vi "ORP电极校准.vi"() -> ()   [LabVIEW 2016, in "斯坦道多参数.lvlib"]
uses:
  <vilib>/Utility/miscctls.llb/LVPointTypeDef.ctl
  <vilib>/Analysis/NI_AALBase.lvlib
  <vilib>/Utility/config.llb/NI_LVConfig.lvlib
panel:
  out "滤波设定":dbl
  in  "刷新按钮":bool
  out "第二点信号值":dbl
  out "第一点信号值":dbl
  out "通讯状态":string
  out "温度":dbl format="%#.2f"
  out "当前信号值":dbl caption="信号值" format="%#.2f"
  in  "校准停止":bool
  in  "校准启动":bool
  out "波形图表":sgl(graph) caption="历史曲线"
  out "第二点校准值":dbl
  out "第一点校准值":dbl
  in  "校准模式":u16(ring) items=["单点校准"]
  out "提示":string
  out "最小值":sgl format="%#.2f"
  out "最大值":sgl format="%#.2f"
  out "mean":dbl caption="均值" format="%#.2f"
  out "standard deviation":dbl caption="标准差" format="%#.2f"
  out "变异系数":dbl format="%#.6f"
  in  "标液1":dbl
  out "当前读取值":dbl caption="测量值" format="%#.2f"
  out "ORP偏移修正值":dbl format="%#.2f"
  # "ORP电极设定"
  # "请选择校准模式:"
  # "℃"
  # "mV"
  # "mV"
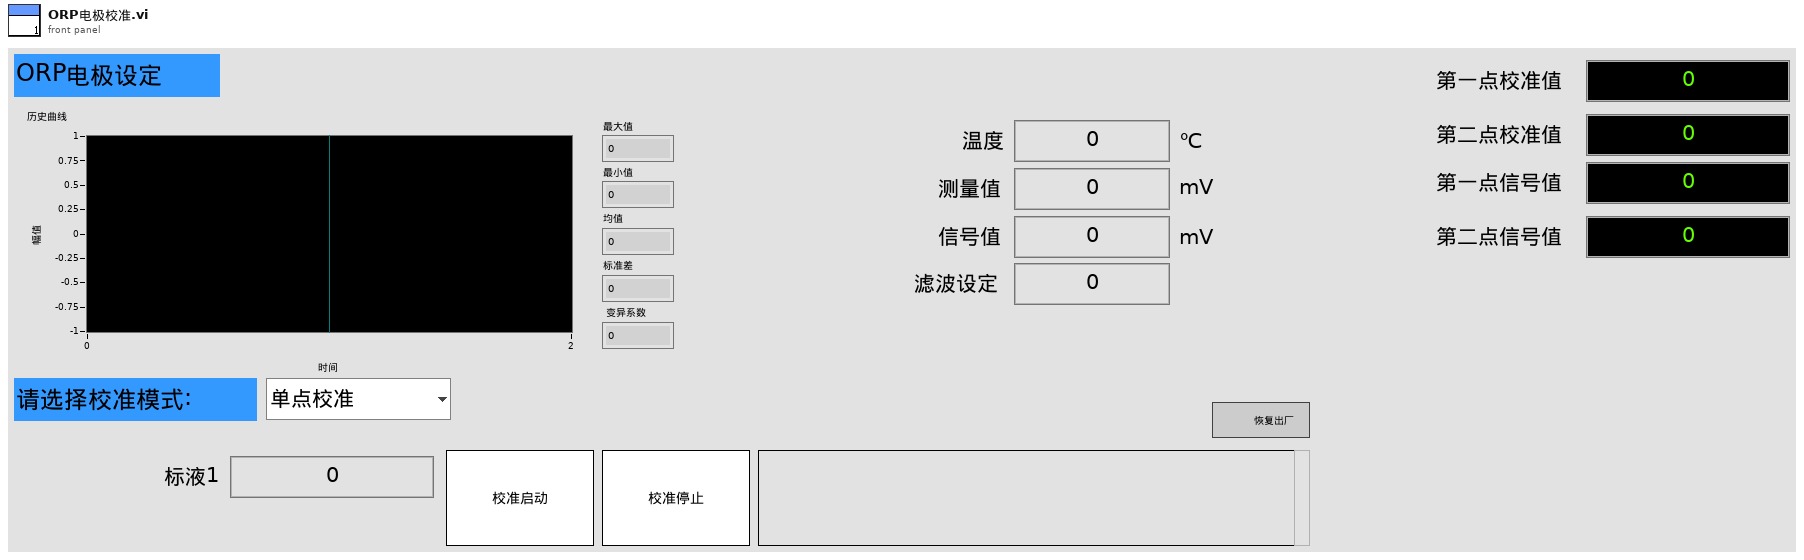
[diagram p1: front panel]
types:
  T1 = typedef "斯坦道多参数.lvlib/通知队列类型.ctl" = enum16{"pH", "DO", "Cond", "Turb", "ORP", "叶绿素a", "藻密度", "COD"}
  T2 = typedef "LVPointTypeDef.ctl" = cluster{"Horizontal":i16, "Vertical":i16}
  T3 = typedef "NI_LVConfig.lvlib/Config Data RefNum.ctl" = refnum<k1>
  T4 = cluster{"电极状态标志":u16, "电极型号标志":u16, "测量值":sgl, "温度测量值":sgl, "信号值":sgl, "温度信号值":sgl, "000AH_NC":sgl, "偏移修正值":sgl, "温度偏移修正值":sgl, "手动温度补偿值":sgl, "命令滤波设定":u16, "温度模式":enum16{"ATC", "MTC"}, "生产批次":u16, "传感器序号":u16, "串口地址":u16, "串口波特率":enum16{"9600", "19200", "115200"}, "串口校验位":enum16{"NONE", "ODD", "EVEN"}, "串口停止位":enum16{"1bit", "2bit"}}
  T5 = enum16{"pH", "DO", "Cond", "Turb", "ORP", "叶绿素a", "藻密度"}
  T6 = enum8{"Enabled", "Disabled", "Disabled and Grayed Out"}
  T7 = cluster{"ph":bool, "DO":bool, "Cond":bool, "Turb":bool, "叶绿素a":bool, "藻密度":bool, "ORP":bool, "COD":bool}
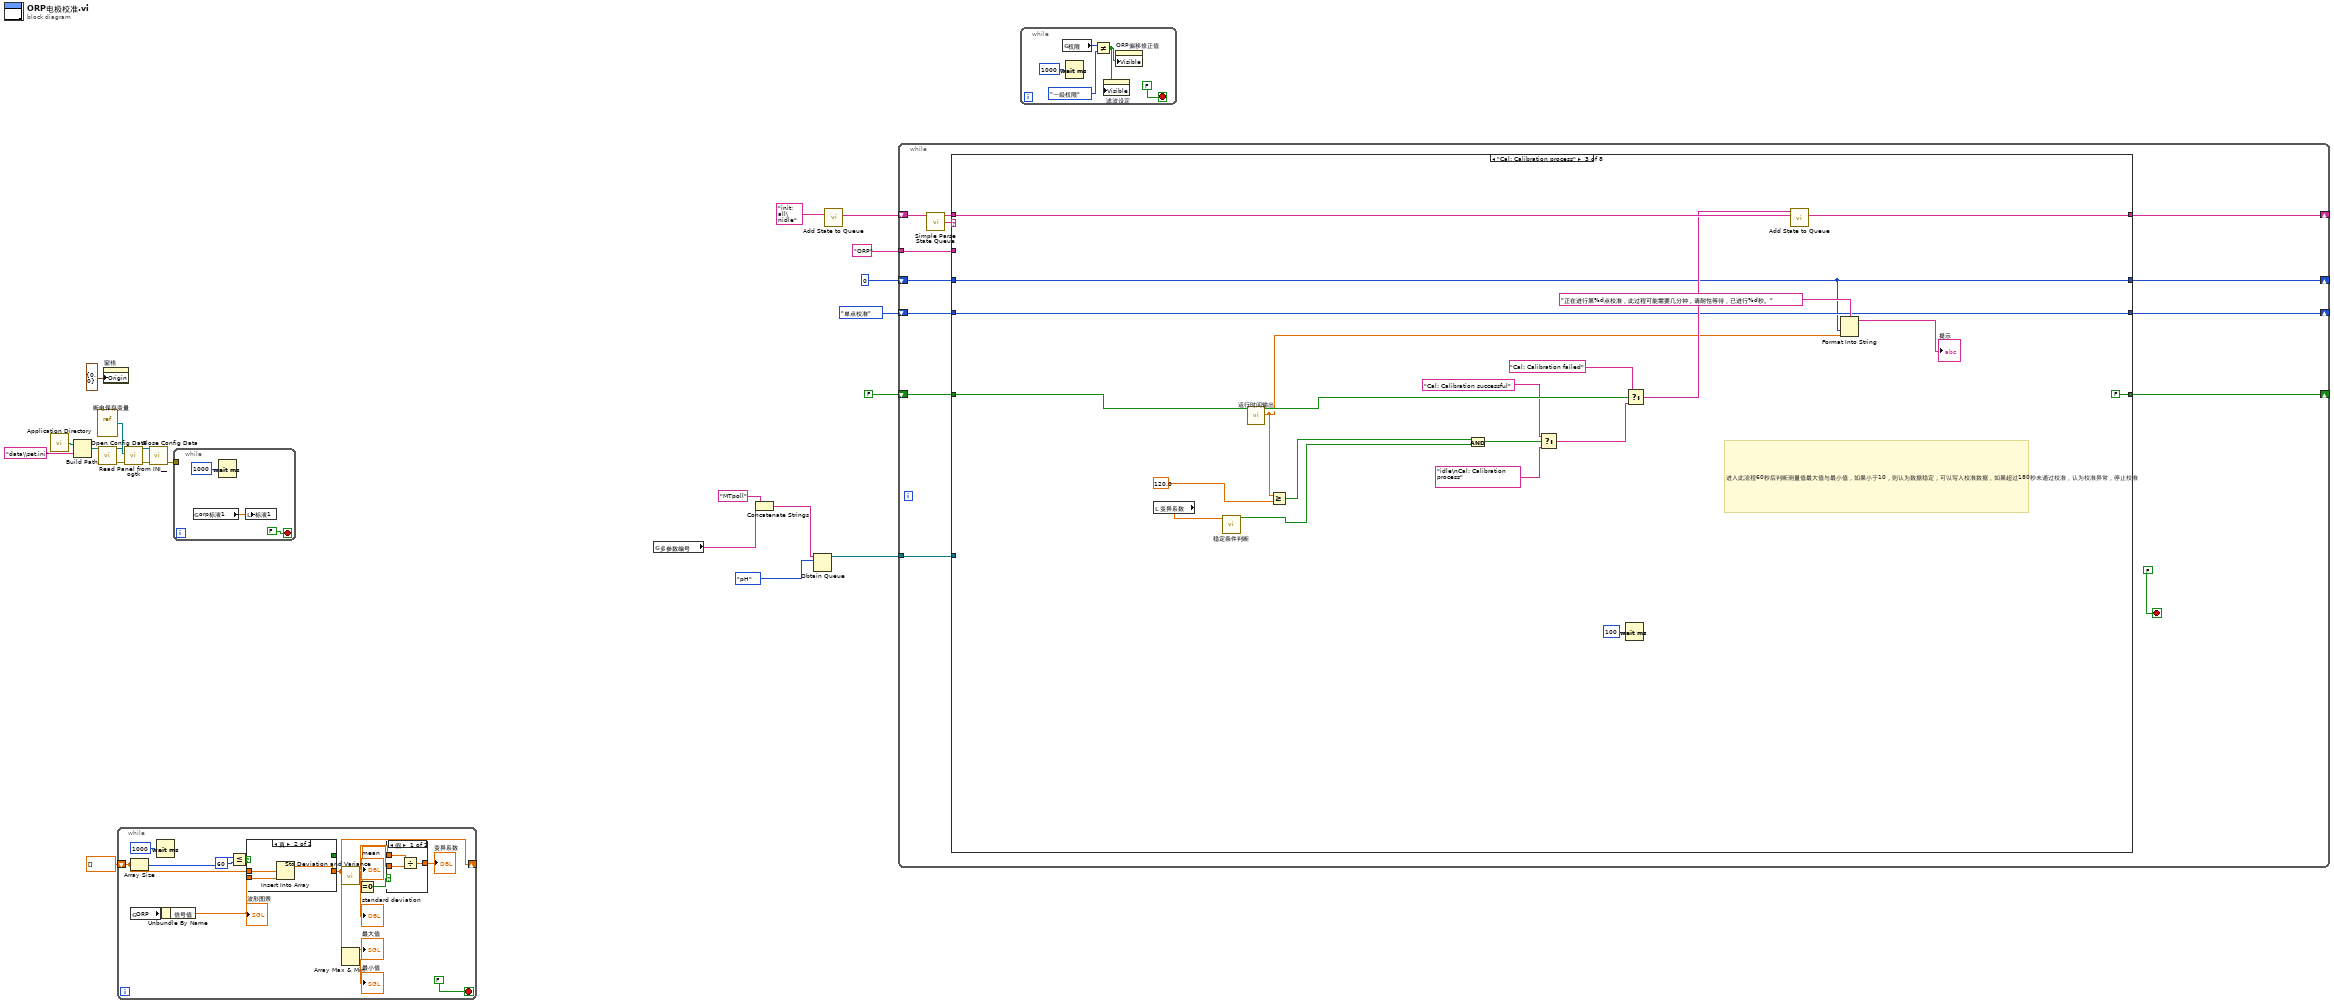
[diagram p0: block diagram]
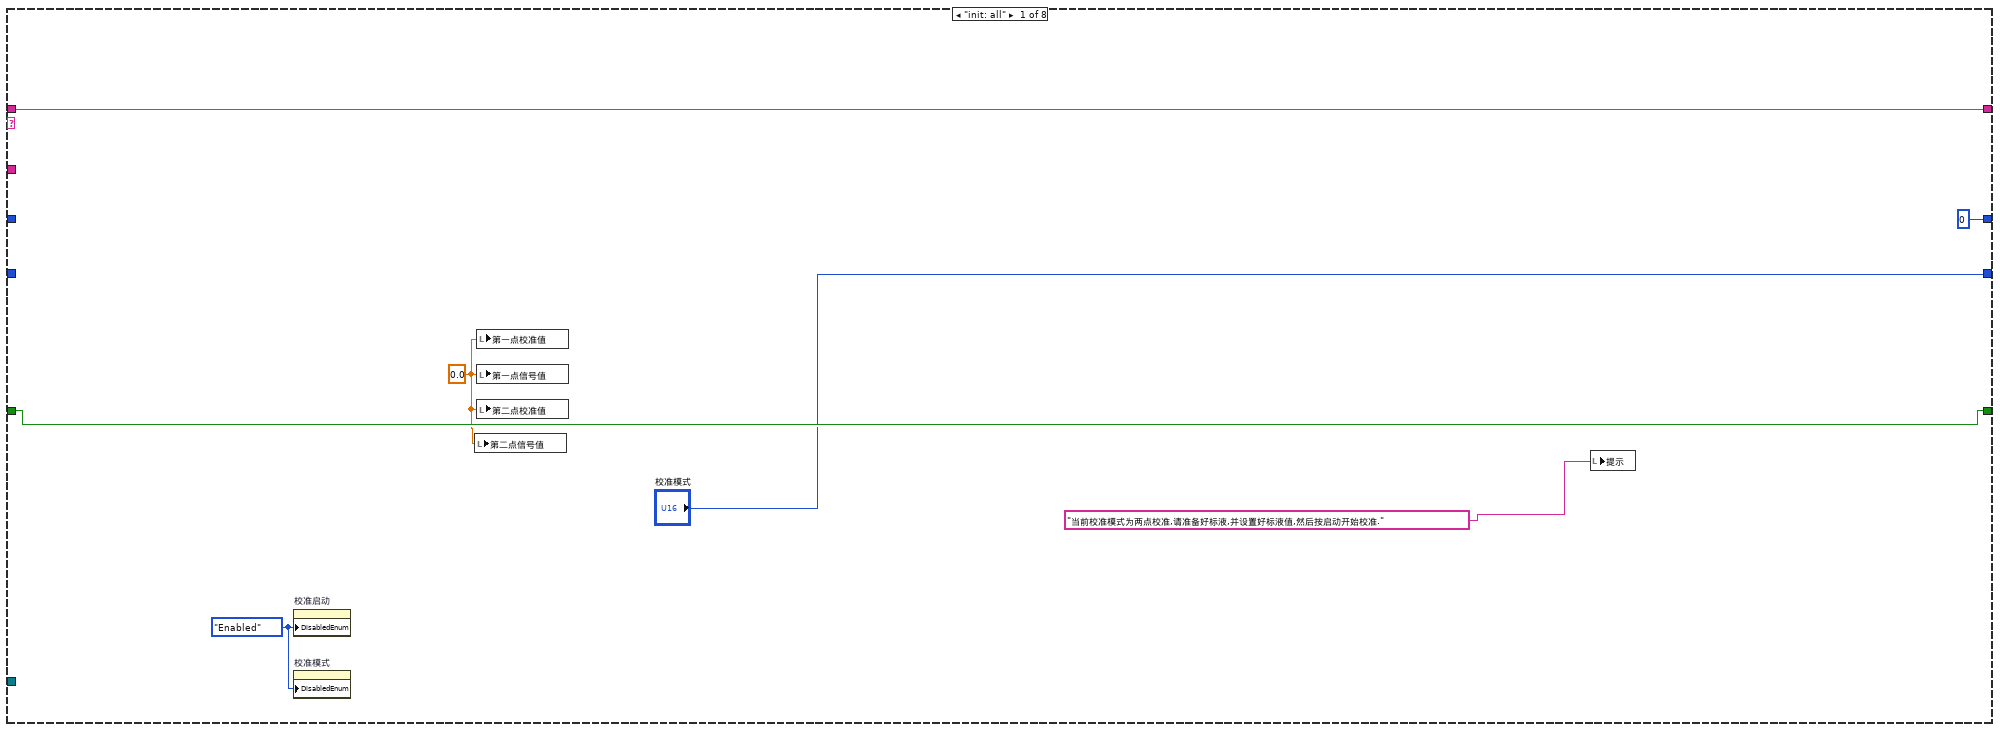
[diagram p2: hidden frame]
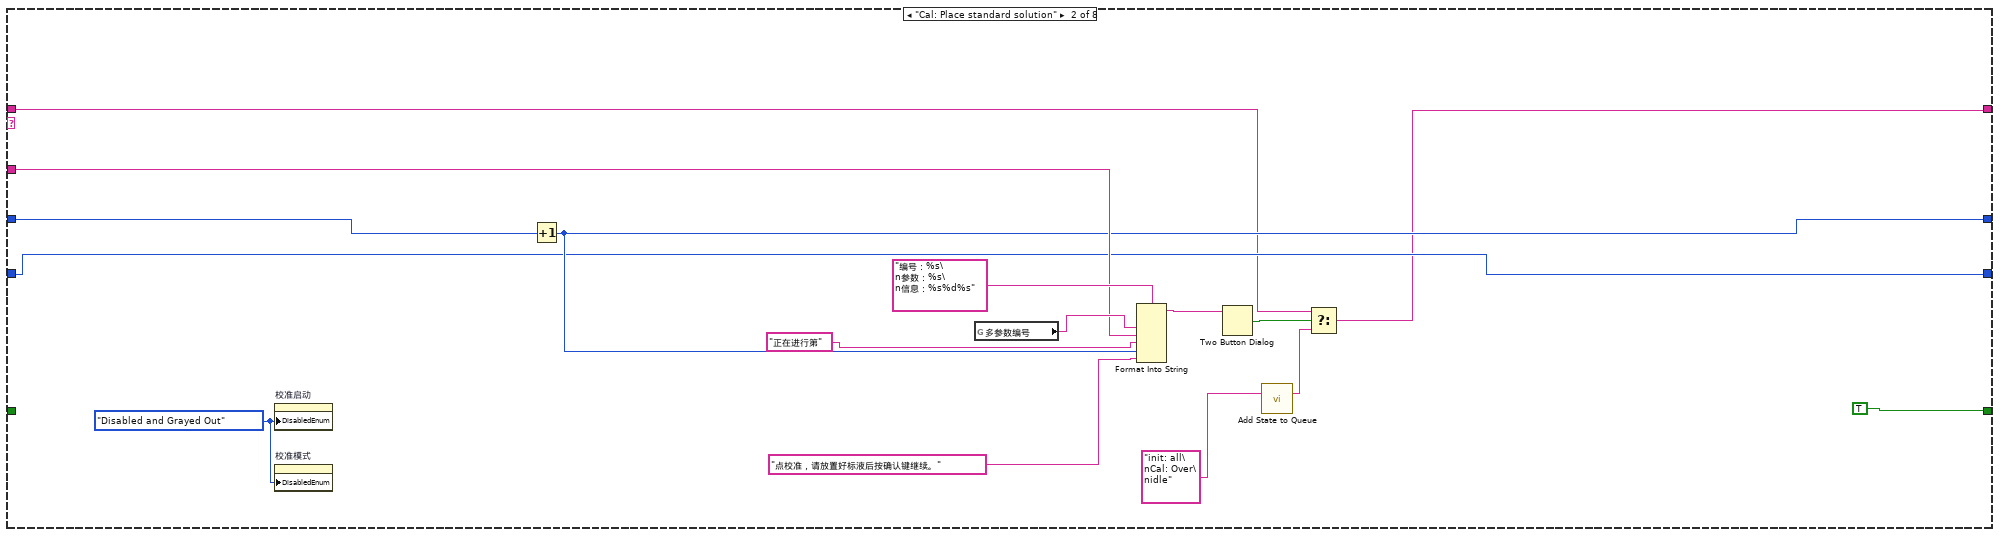
[diagram p3: hidden frame]
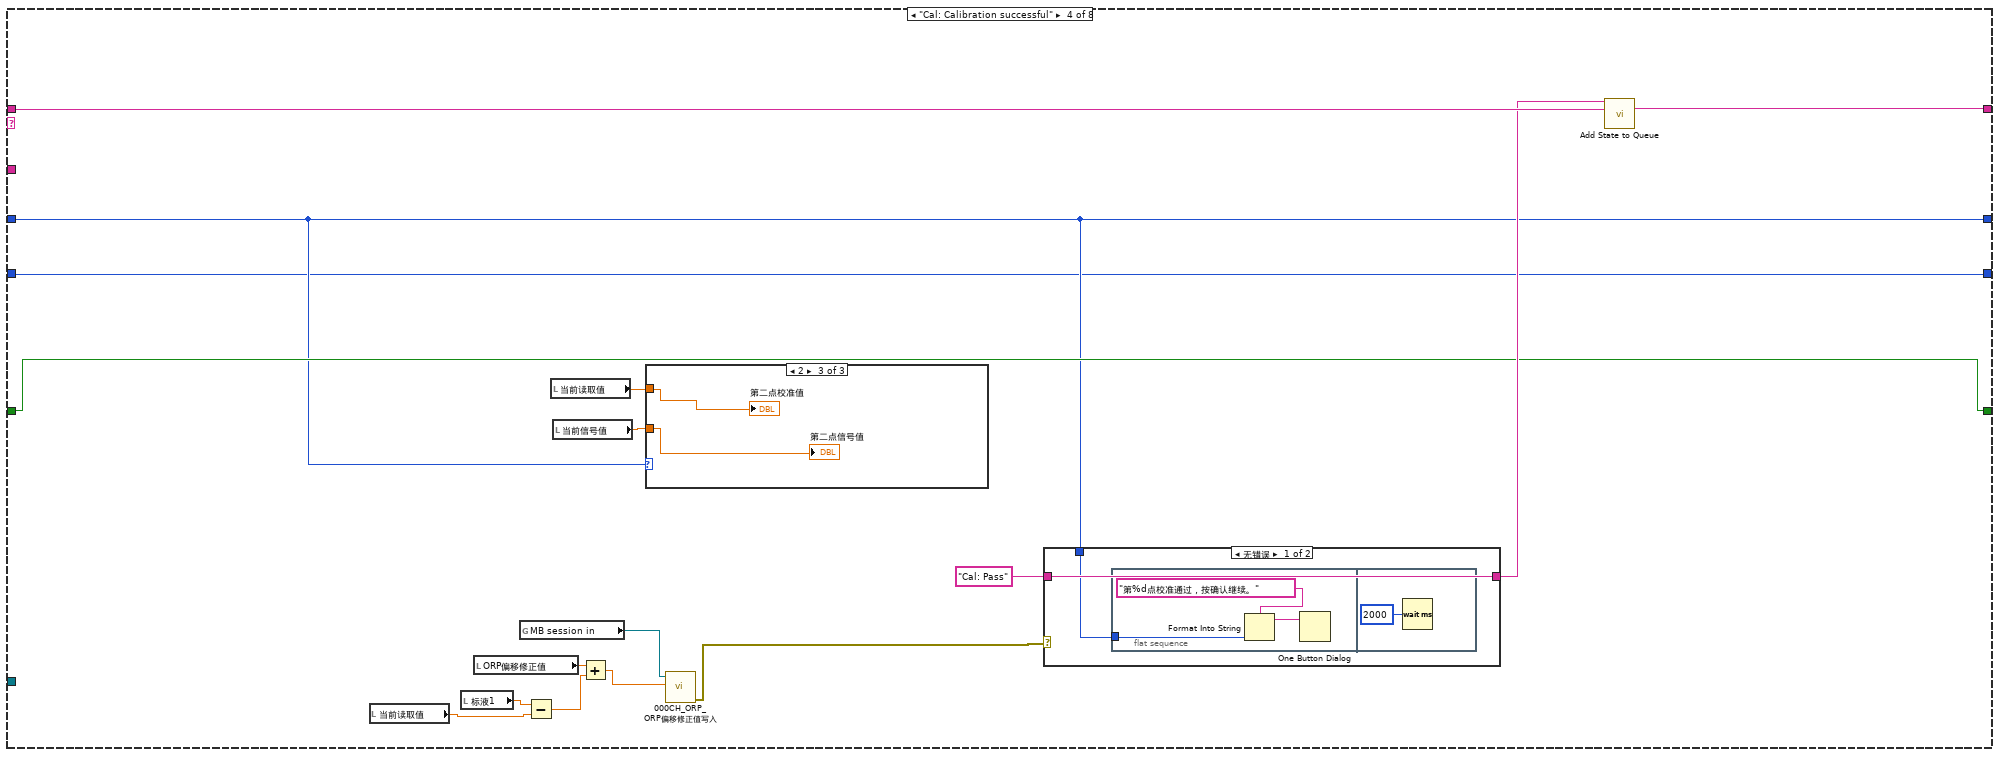
[diagram p4: hidden frame]
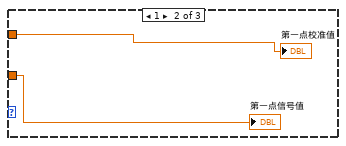
[diagram p6: hidden frame]
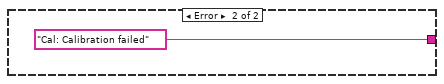
[diagram p7: hidden frame]
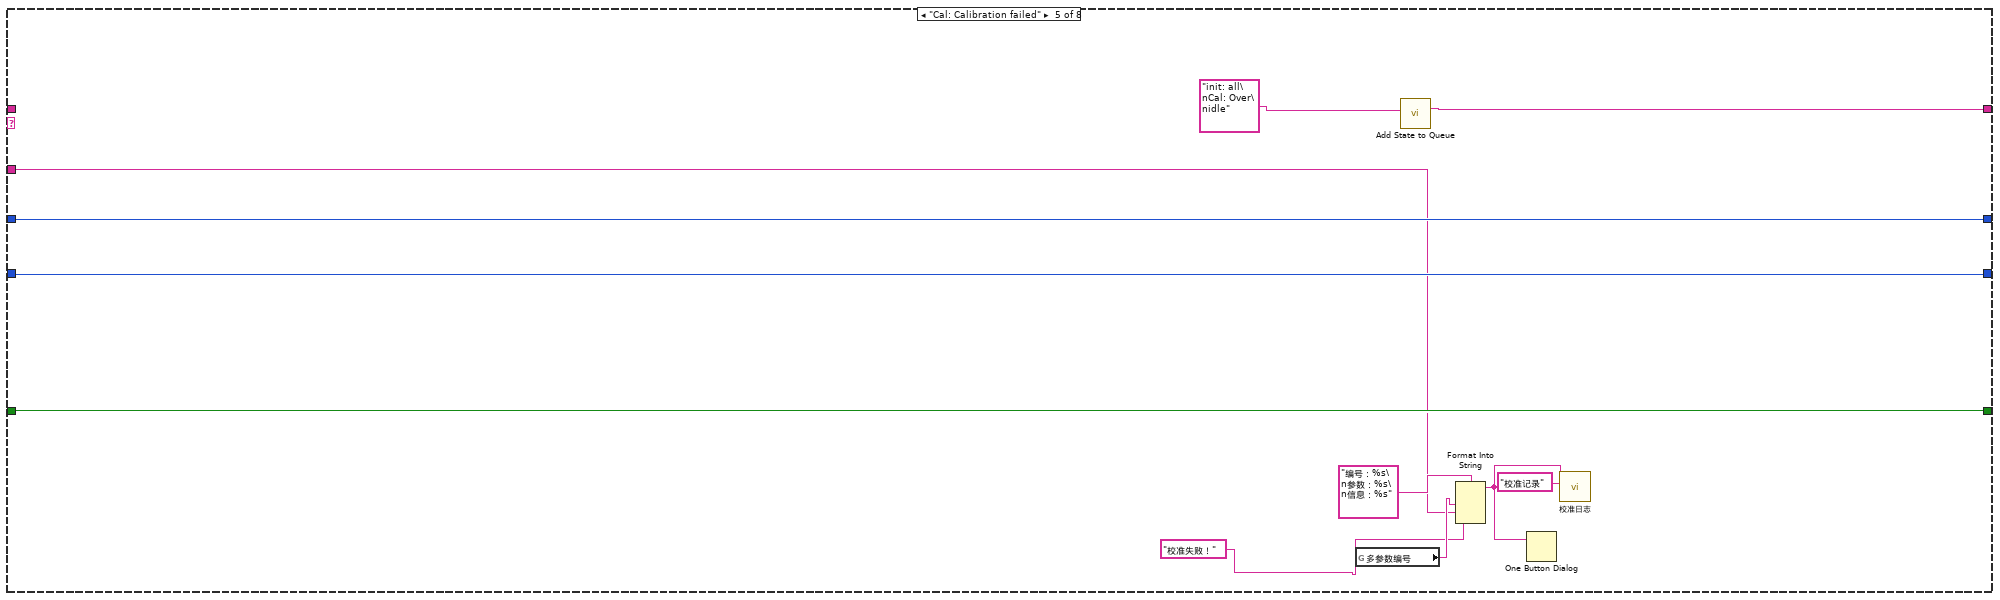
[diagram p8: hidden frame]
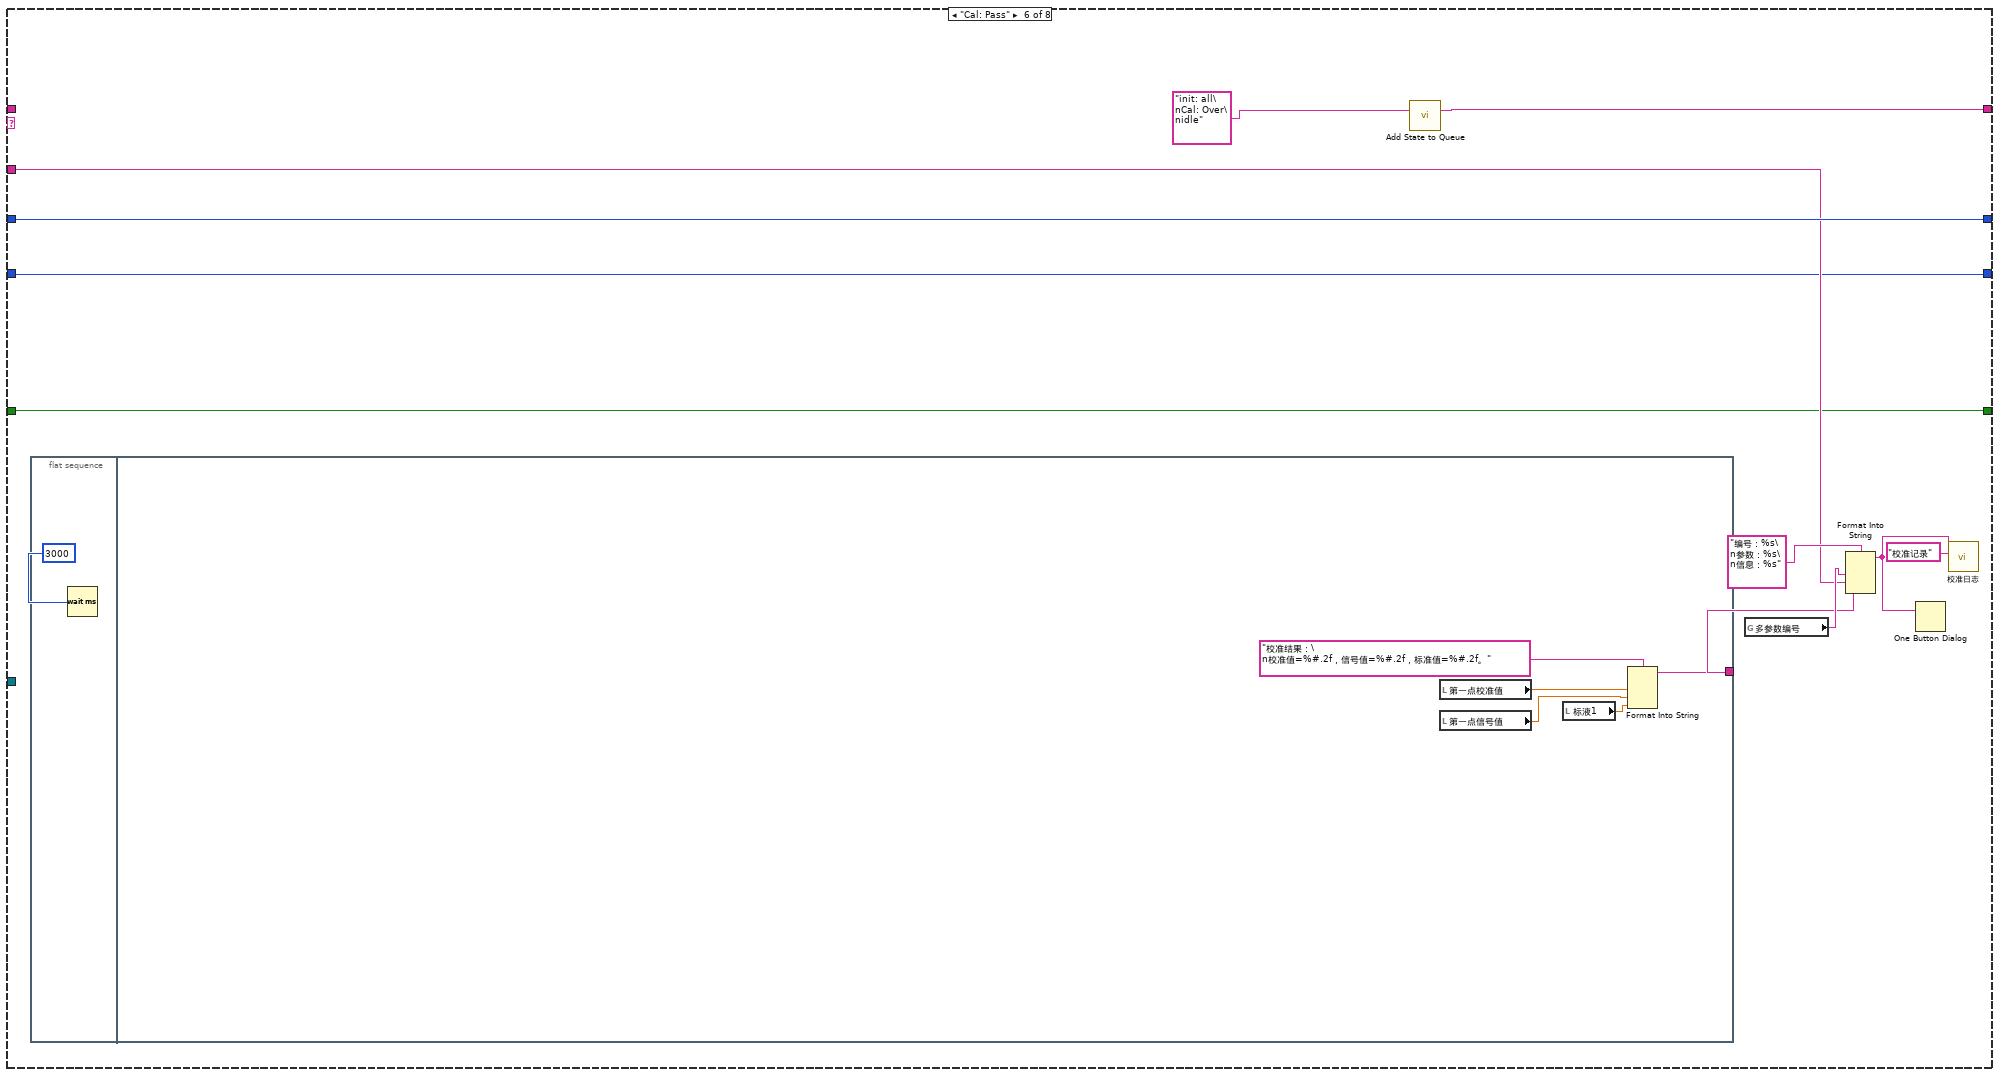
[diagram p9: hidden frame]
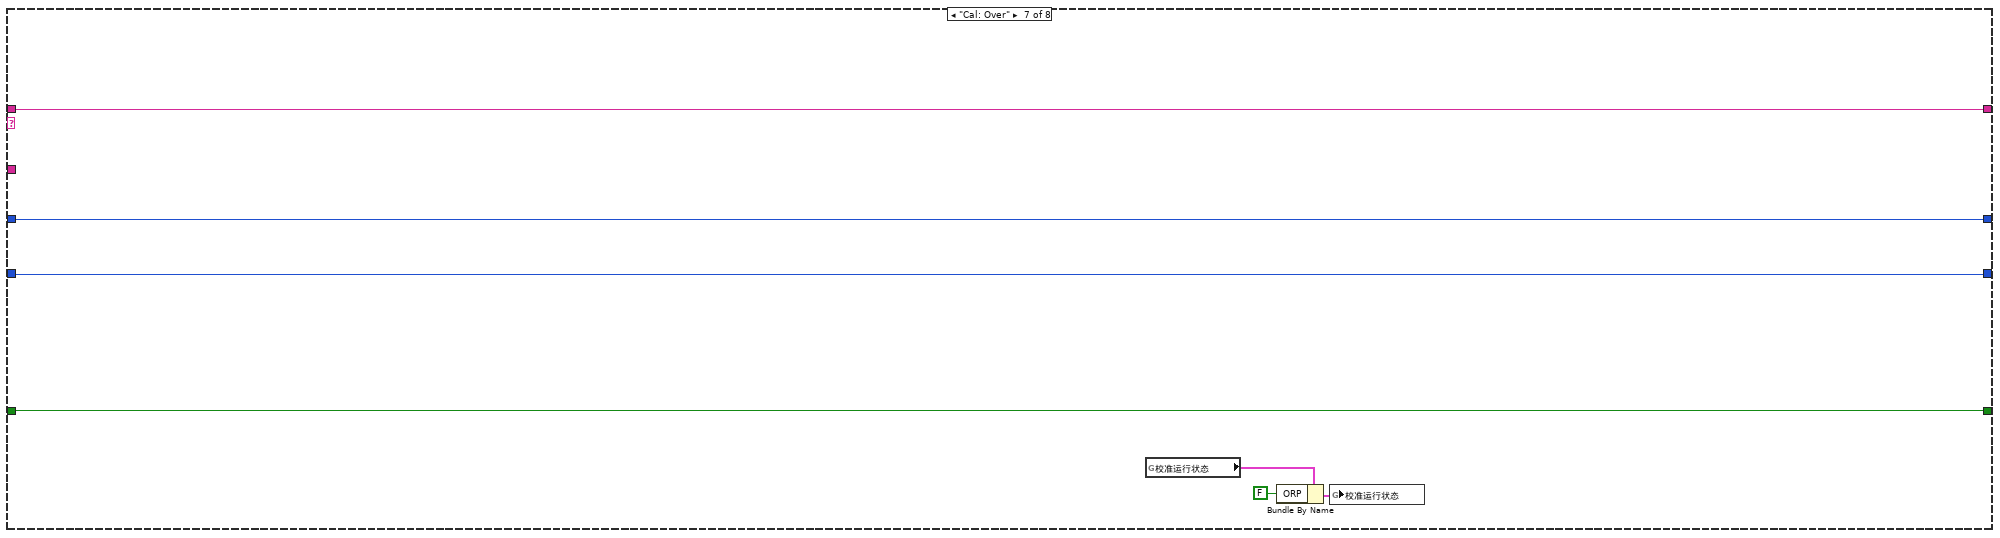
[diagram p10: hidden frame]
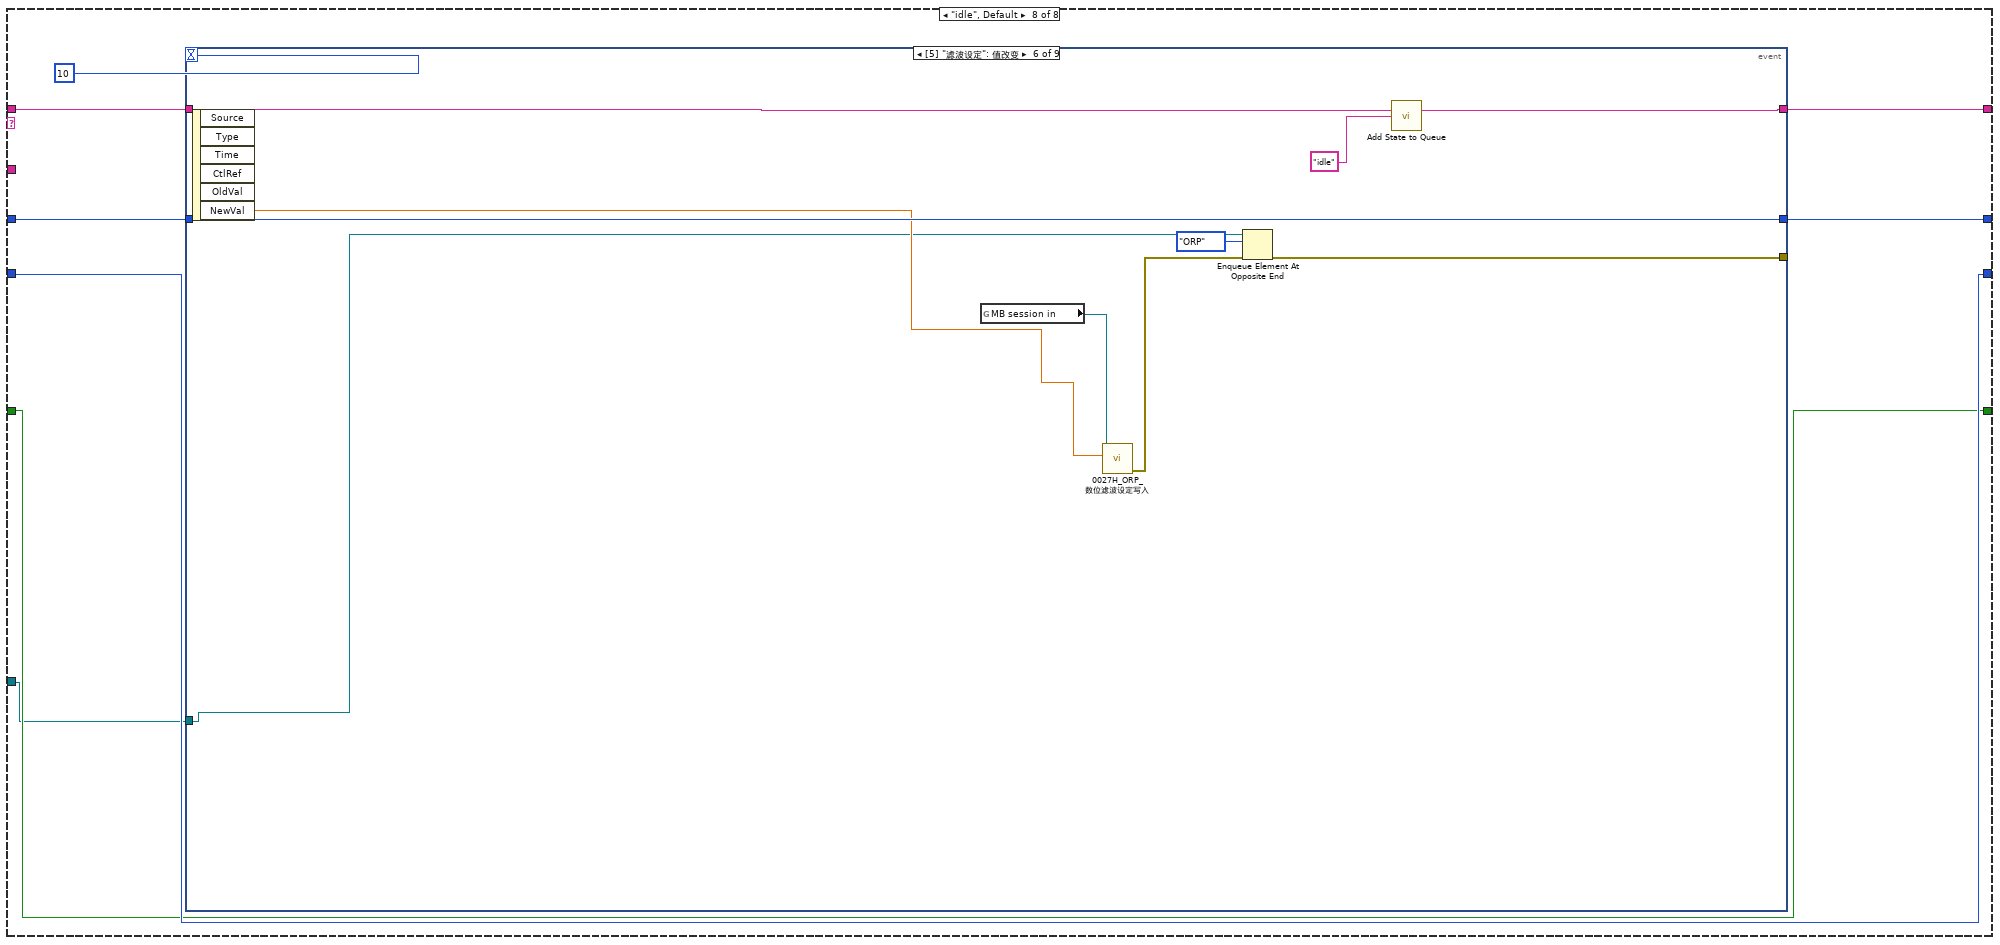
[diagram p11: hidden frame]
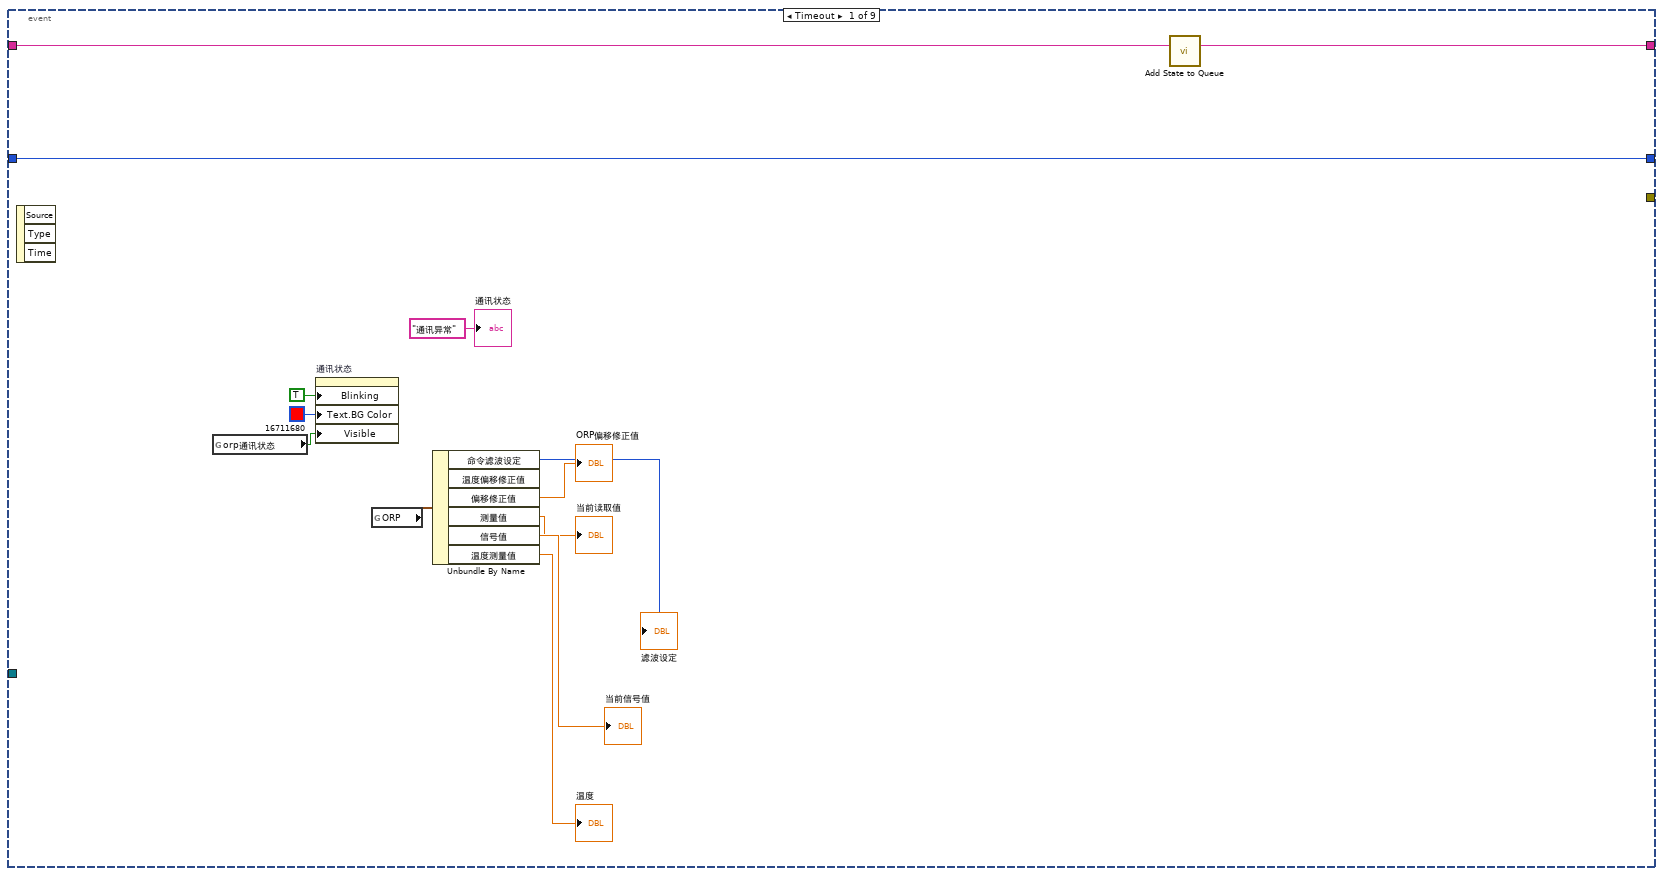
[diagram p12: hidden frame]
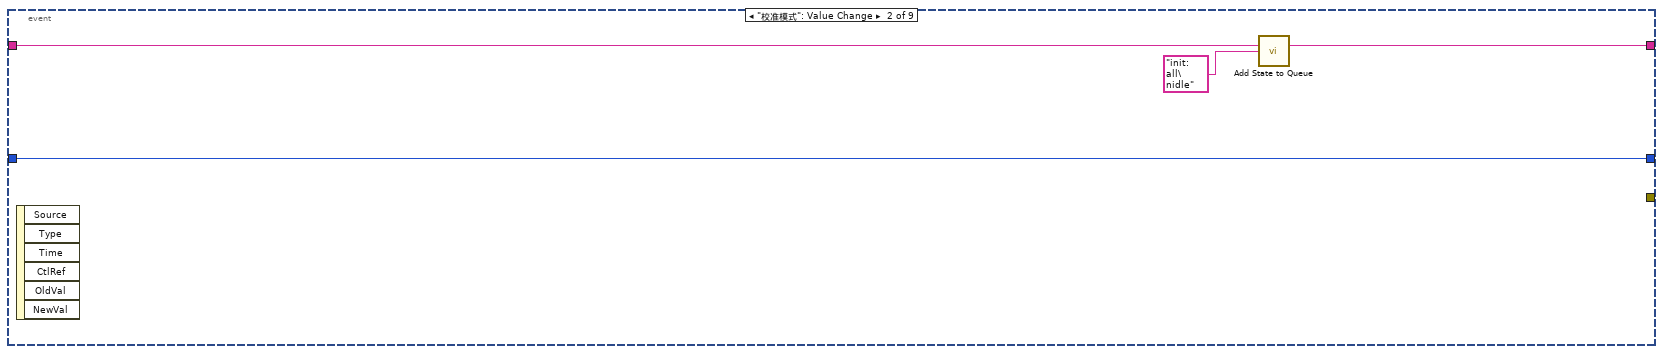
[diagram p13: hidden frame]
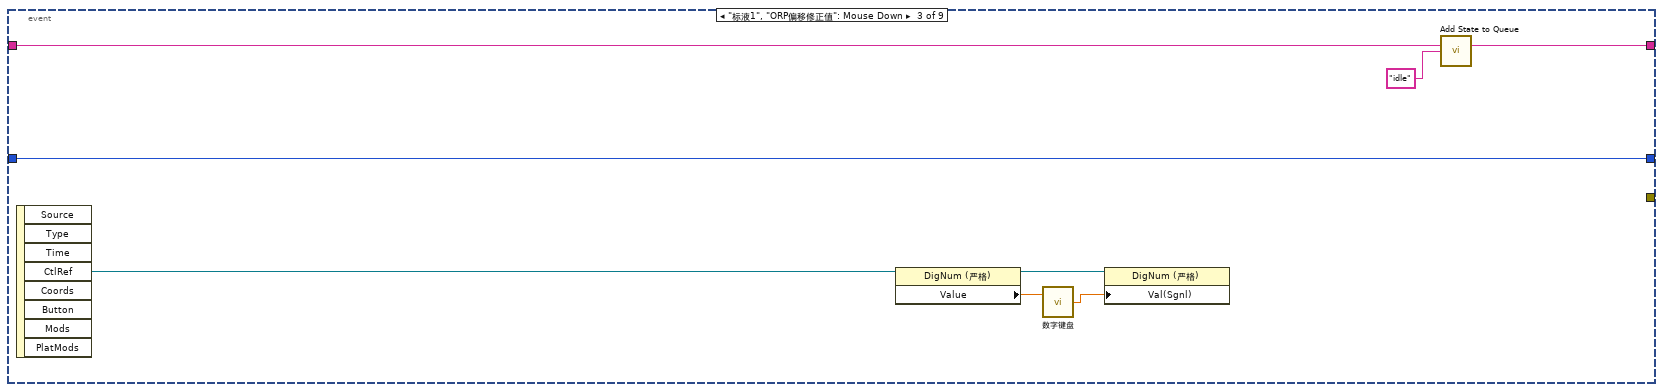
[diagram p14: hidden frame]
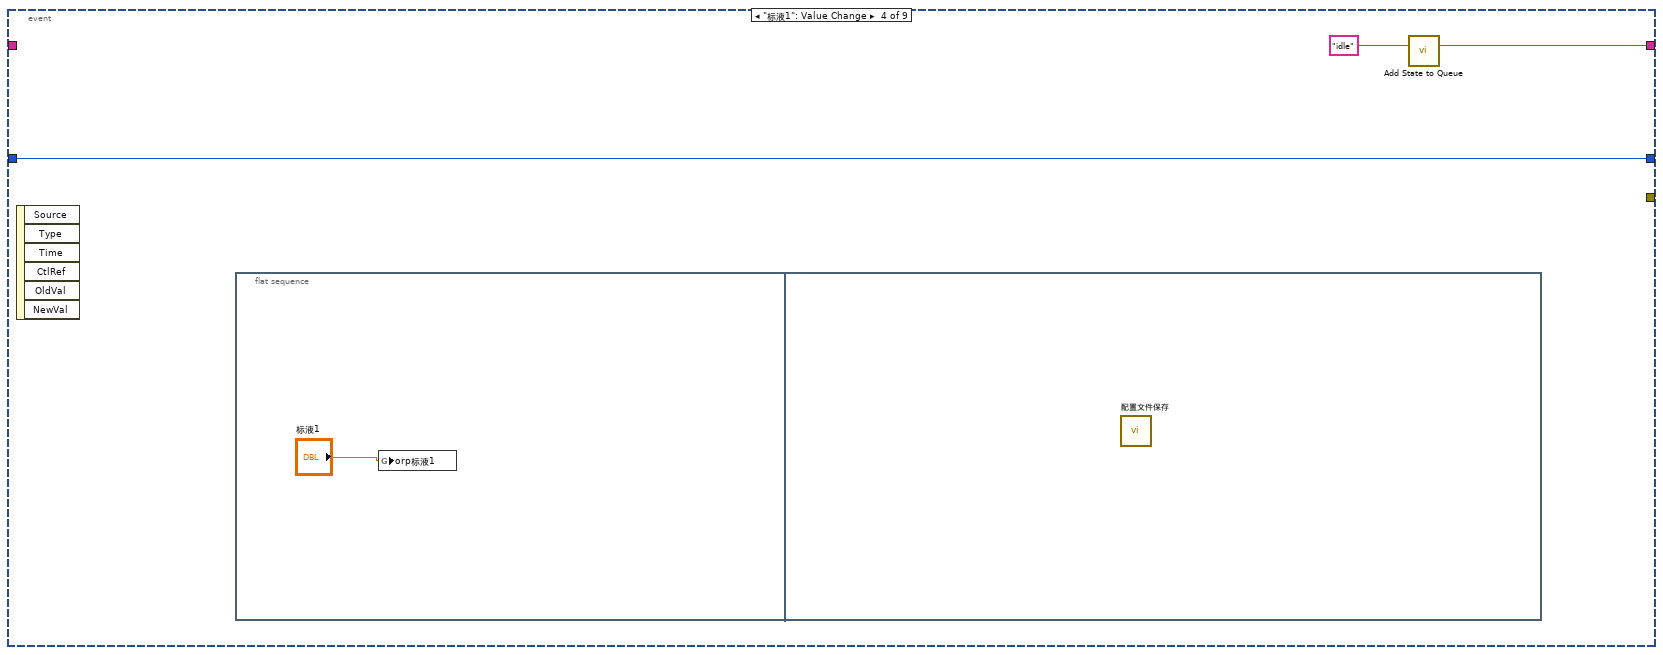
[diagram p15: hidden frame]
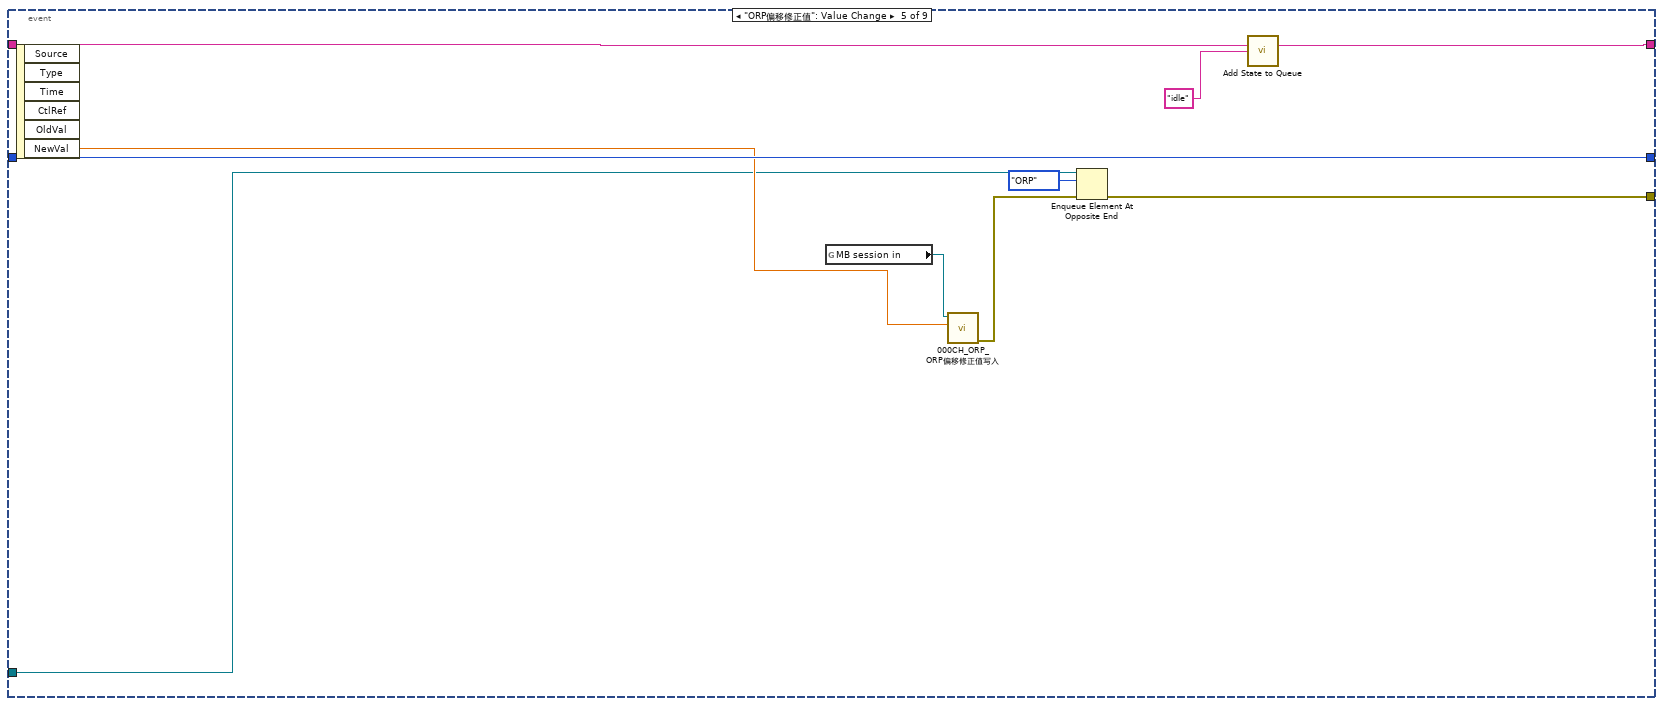
[diagram p16: hidden frame]
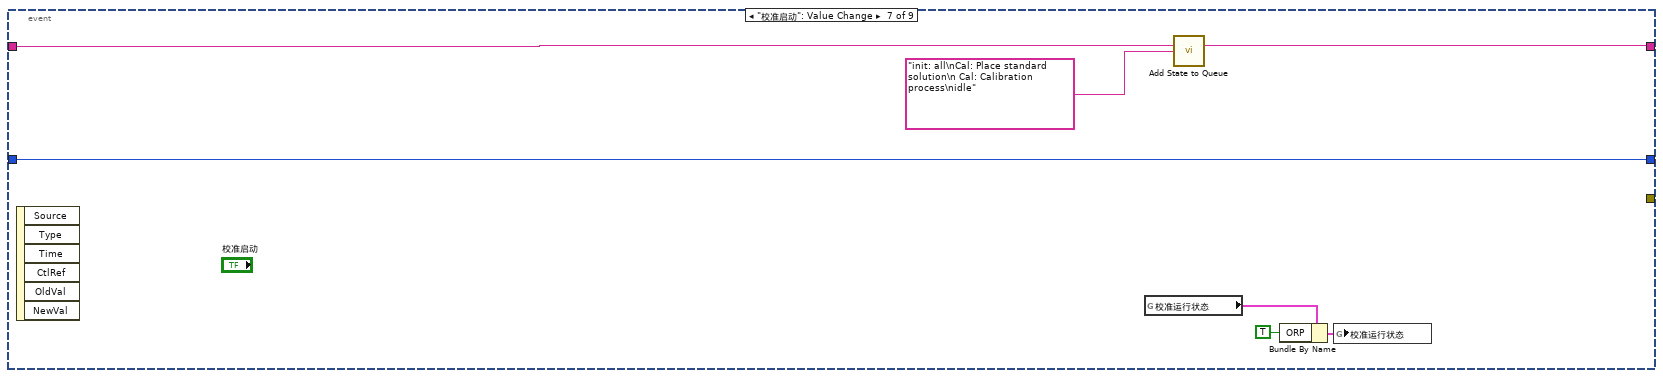
[diagram p17: hidden frame]
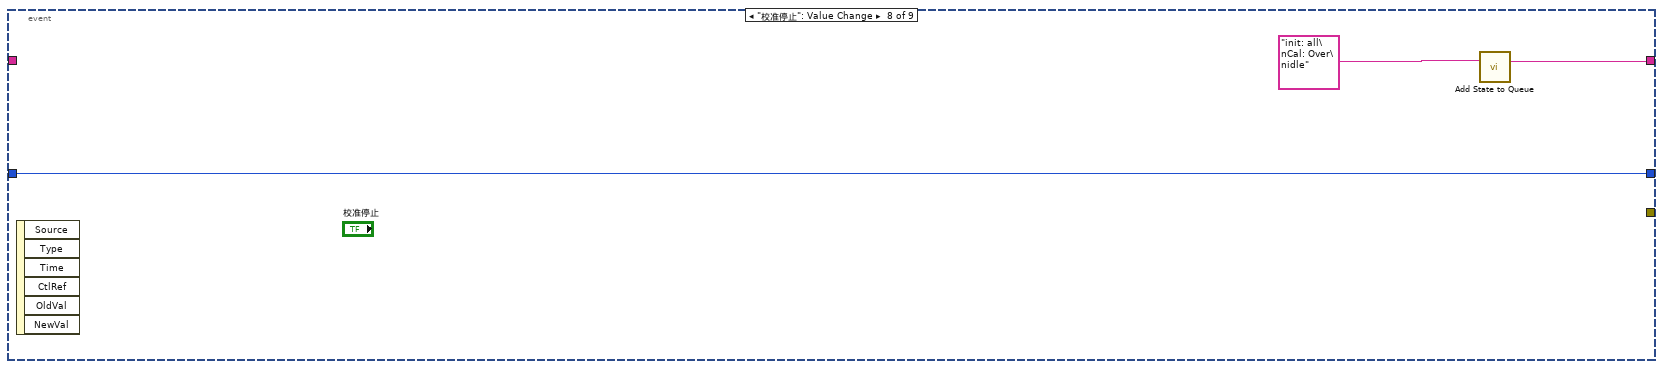
[diagram p18: hidden frame]
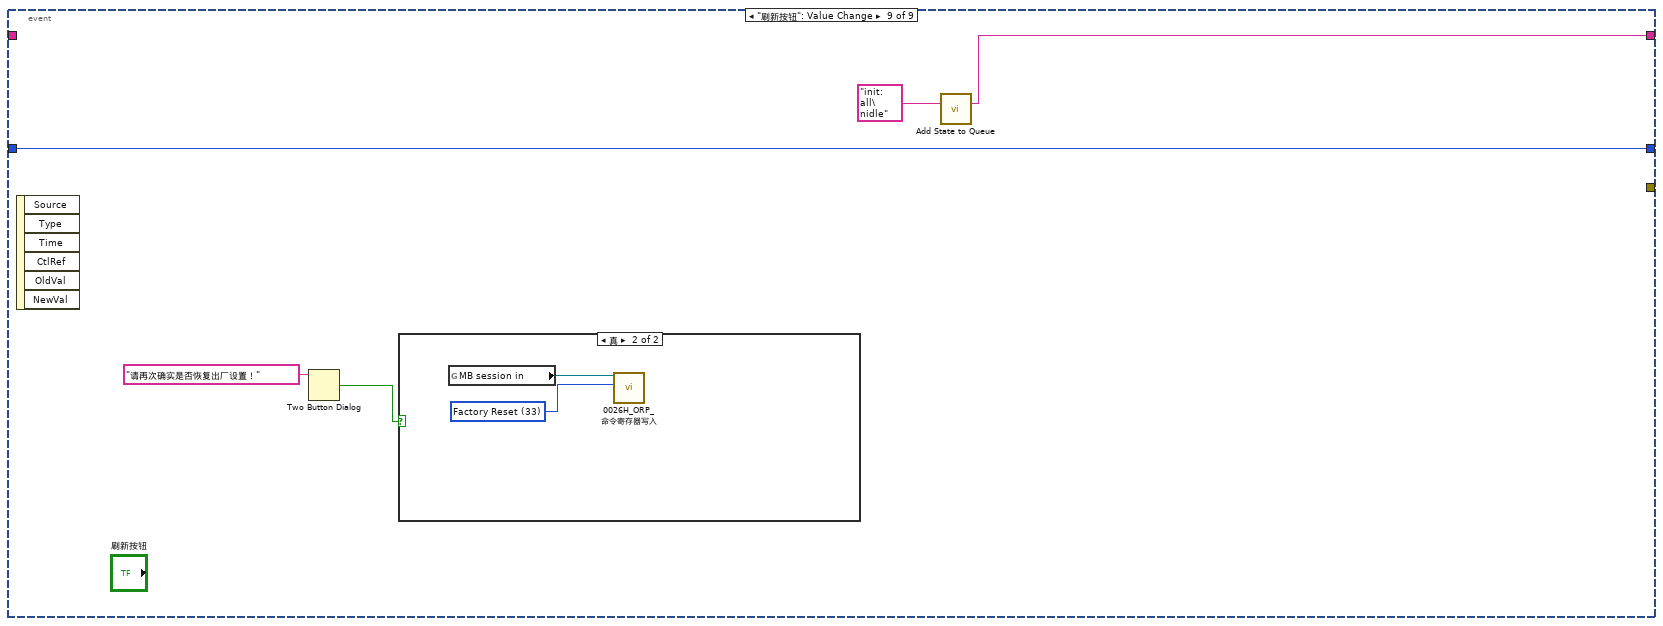
[diagram p19: hidden frame]
diagram:
  n1 = call <vilib>:"Application Directory.vi"() -> ("Application Directory"=w11:path)
  n2 = Build Path(base path=w11, name or relative path="data\\set.ini" ("名称或相对路径")) -> (appended path=w12:path)
  n3 = vi-ref "断电保存变量.vi"() -> (w14:refnum<vi>)
  n4 = call <vilib>:"Open Config Data.vi"("configuration file path"=w12) -> ("error out"=w8:errorcluster, "refnum"=w7:T3)  [unwired: 8 in, 1 out]
  n5 = property on="窗格" class="Pane"("Origin"=T2 {"Horizontal"=0, "Vertical"=0} ("原点")) -> ()  [unwired: 2 in, 2 out]
  n6 = while {
    shift-right: [w26] -> _
    shift-left: sgl[] [] -> [w33]
    stop <- FALSE stop-if-true
    n7 = Array Size(array=w33) -> (size(s)=w35:i32)
    n8 = global read "国弘过程全局变量.vi" "ORP"() -> (w27:T4)
    n9 = Wait (ms)(milliseconds to wait=u32 1000 ("等待时间（毫秒）")) -> ()  [unwired: 1 out]
    n10 = Unbundle By Name(w27) -> ("信号值"=w23:sgl)
    "波形图表" <- w23
    n11 = Less Or Equal?(x=w35, y=60) -> (x <= y?=w34:bool)
    n12 = case shown="真" w34 {
      tunnel: w33 -> [w46 w49]
      tunnel: w23 -> [w44 w48]
      tunnel: [w42 w47] -> w26
      tunnel: [TRUE _] -> _
      frame False {
        n13 = Replace Array Subset(array=w46, new element=w44) -> (w45:sgl[])  [unwired: 1 in]
        n14 = Rotate 1D Array(1:w45, 2:-1 ("n")) -> (0:w42:sgl[])
      }
      frame True {
        n15 = Insert Into Array(array=w49, new element=w48) -> (w47:sgl[])  [unwired: 1 in]
      }
    }
    n16 = call <vilib>:"Std Deviation and Variance.vi"("X"=w26) -> ("mean"=w31:dbl, "standard deviation"=w30:dbl)  [unwired: 1 in, 1 out]
    "mean" <- w31
    "standard deviation" <- w30
    n17 = Array Max & Min(array=w26) -> (max value=→"最大值":sgl, min value=→"最小值":sgl)  [unwired: 2 out]
    n18 = Equal To 0?(x=w31) -> (x = 0?=w32:bool)
    n19 = case shown="假" w32 {
      tunnel: w30 -> [w40 _]
      tunnel: [w39 _] -> w29
      tunnel: w31 -> [w38 _]
      frame False {
        n20 = Divide(x=w40, y=w38) -> (x/y=w39:dbl)
      }
      frame True {
      }
    }
    "变异系数" <- w29
  }
  n21 = call <userlib>:"Read Panel from INI__ogtk.vi"("error in (no error)"=w8, "VI ref"=w14, "refnum"=w7) -> ("error out"=w10:errorcluster, "refnum out"=w9:T3)  [unwired: 7 in]
  n22 = call <vilib>:"Close Config Data.vi"("error in (no error)"=w10, "refnum"=w9) -> ("error out"=w6:errorcluster)  [unwired: 8 in, 1 out]
  n23 = while {
    tunnel: w6 -> [_]
    stop <- FALSE stop-if-true
    n24 = global read "断电保存变量.vi" "orp标液1"() -> (w50:dbl)
    n25 = Wait (ms)(milliseconds to wait=u32 1000 ("等待时间（毫秒）")) -> ()  [unwired: 1 out]
    n26 = local write "标液1"(w50) -> ()
  }
  n27 = global read "多参数全局变量.vi" "多参数编号"() -> (w3:string)
  n28 = Concatenate Strings("MTpoll" ("名称（未命名）"), w3) -> (w4:string)
  n29 = Obtain Queue(name (unnamed)=w4, element data type=通知队列类型."pH" ("枚举")) -> (queue out=w2:refnum<queue>)  [unwired: 3 in, 2 out]
  n30 = call "Add State to Queue.vi"("State(s) In (\"\")"="init: all\nidle" ("State(s) In (\"\")")) -> ("States Out"=w19:string)  [unwired: 14 in]
  n31 = while {
    shift-right: [w61] -> _
    shift-left: w19 -> [w65]
    shift-right: [w58] -> _
    shift-left: 0 -> [w60]
    tunnel: "ORP" ("State(s) In (\"\")") -> [w59]
    shift-right: [w56] -> _
    shift-left: enum16{"单点校准"}."单点校准" ("校准模式") -> [w57]
    shift-right: [w54] -> _
    shift-left: FALSE -> [w55]
    tunnel: w2 -> [w53]
    stop <- FALSE stop-if-true
    n32 = call "Simple Parse State Queue.vi"("State Queue"=w65) -> ("Remain States"=w62:string, "Next State"=w63:string)  [unwired: 13 in]
    n33 = case shown="\"Cal: Calibration process\"" w63 {
      tunnel: w62 -> [w72 w76 w108 w124 _ _ w168 w179]
      tunnel: [w72 w75 w107 w123 w144 w149 w168 w178] -> w61
      tunnel: w60 -> [_ w84 w93 w118 w147 w158 w165 w176]
      tunnel: w59 -> [_ w85 _ _ w138 w154 _ _]
      tunnel: [0 w82 w93 w118 w147 w158 w165 w177] -> w58
      tunnel: w57 -> [_ w81 w94 w117 w146 w150 w166 w175]
      tunnel: ["校准模式" w81 w94 w117 w146 w150 w166 w175] -> w56
      tunnel: w55 -> [w69 _ w96 w119 w145 w153 w167 w173]
      tunnel: [w69 TRUE FALSE w119 w145 w153 w167 w173] -> w54
      tunnel: w53 -> [_ _ _ _ _ _ _ w172]
      frame "init: all" {
        w67 = T6."Enabled" ("禁用")
        w66 = 0.0 ("第一点校准值")
        n34 = property on="校准启动" class="Bool"("DisabledEnum"=w67) -> ()  [unwired: 2 in, 2 out]
        n35 = property on="校准模式" class="Ring (严格)"("DisabledEnum"=w67) -> ()  [unwired: 2 in, 2 out]
        n36 = local write "第二点信号值"(w66) -> ()
        n37 = local write "第一点校准值"(w66) -> ()
        n38 = local write "第一点信号值"(w66) -> ()
        n39 = local write "第二点校准值"(w66) -> ()
        n40 = local write "提示"("当前校准模式为两点校准,请准备好标液,并设置好标液值,然后按启动开始校准." ("提示")) -> ()
      }
      frame "Cal: Place standard solution" {
        w74 = T6."Disabled and Grayed Out" ("禁用")
        n41 = property on="校准启动" class="Bool"("DisabledEnum"=w74) -> ()  [unwired: 2 in, 2 out]
        n42 = property on="校准模式" class="Ring (严格)"("DisabledEnum"=w74) -> ()  [unwired: 2 in, 2 out]
        n43 = Increment(x=w84) -> (x+1=w82:i32)
        n44 = global read "多参数全局变量.vi" "多参数编号"() -> (w87:string)
        n45 = Format Into String(format string="编号：%s\n参数：%s\n信息：%s%d%s" ("格式字符串"), w87, w85, "正在进行第" ("消息"), w82, "点校准，请放置好标液后按确认键继续。" ("消息")) -> (resulting string=w79:string)  [unwired: 2 in, 1 out]
        n46 = Two Button Dialog(message=w79) -> (T button?=w78:bool)  [unwired: 2 in]
        n47 = call "Add State to Queue.vi"("State(s) In (\"\")"="init: all\nCal: Over\nidle" ("State(s) In (\"\")")) -> ("States Out"=w77:string)  [unwired: 14 in]
        n48 = Select(t=w76, s=w78, f=w77) -> (s? t:f=w75:string)
      }
      frame "Cal: Calibration process" {
        # "进入此流程60秒后判断测量值最大值与最小值，如果小于10，则认为数据稳定，可以写入校准数据，如果超过180秒未通过校准，认为校准异常，停止校准"
        n49 = local read "变异系数"() -> (w90:dbl)
        n50 = call "稳定条件判断.vi"("变异系数"=w90) -> ("布尔"=w89:bool)  [unwired: 10 in]
        n51 = call "运行时间输出.vi"("初始化"=w96) -> ("Elapsed Time (s)"=w92:dbl, "Time has Elapsed"=w109:bool)  [unwired: 9 in]
        n52 = Greater Or Equal?(x=w92, y=120.0) -> (x >= y?=w104:bool)
        n53 = And(x=w104, y=w89) -> (x .and. y?=w101:bool)
        n54 = Select(t="Cal: Calibration successful" ("State(s) In (\"\")"), s=w101, f="idle\nCal: Calibration process" ("State(s) In (\"\")")) -> (s? t:f=w100:string)
        n55 = Wait (ms)(milliseconds to wait=u32 100 ("等待时间（毫秒）")) -> ()  [unwired: 1 out]
        n56 = Select(t="Cal: Calibration failed" ("State(s) In (\"\")"), s=w109, f=w100) -> (s? t:f=w99:string)
        n57 = call "Add State to Queue.vi"("State(s) In Front (\"\")"=w99, "State(s) In (\"\")"=w108) -> ("States Out"=w107:string)  [unwired: 13 in]
        n58 = Format Into String(format string="正在进行第%d点校准，此过程可能需要几分钟，请耐性等待，已进行%d秒。" ("格式字符串"), w93, w92) -> (resulting string=→"提示":string)  [unwired: 2 in, 1 out]
      }
      frame "Cal: Calibration successful" {
        n59 = local read "当前读取值"() -> (w113:dbl)
        n60 = local read "标液1"() -> (w116:dbl)
        n61 = local read "ORP偏移修正值"() -> (w114:dbl)
        n62 = global read "多参数全局变量.vi" "MB session in"() -> (w112:refnum<class "MB_Master.lvclass">)
        n63 = Subtract(x=w116, y=w113) -> (x-y=w115:dbl)
        n64 = local read "当前读取值"() -> (w120:dbl)
        n65 = local read "当前信号值"() -> (w121:dbl)
        n66 = Add(x=w114, y=w115) -> (x+y=w111:dbl)
        n67 = case shown="2" w118 {
          tunnel: w121 -> [_ w127 w129]
          tunnel: w120 -> [_ w126 w128]
          frame 0, Default {
          }
          frame 1 {
            "第一点信号值" <- w127
            "第一点校准值" <- w126
          }
          frame 2 {
            "第二点信号值" <- w129
            "第二点校准值" <- w128
          }
        }
        n68 = call "000CH_ORP_ORP偏移修正值写入.vi"("数值"=w111, "MB session in"=w112) -> ("error out"=w110:errorcluster)  [unwired: 8 in, 1 out]
        n69 = case shown="无错误" w110 {
          tunnel: "Cal: Pass" ("State(s) In (\"\")") -> [w131 _]
          tunnel: [w131 "Cal: Calibration failed" ("State(s) In (\"\")")] -> w122
          tunnel: w118 -> [w130 _]
          frame No Error {
            n70 = flat-sequence {
              tunnel: w130 -> [w132]
              frame #0 {
                n71 = Format Into String(format string="第%d点校准通过，按确认继续。" ("格式字符串"), w132) -> (resulting string=w134:string)  [unwired: 2 in, 1 out]
                n72 = One Button Dialog(message=w134) -> ()  [unwired: 1 in, 1 out]
              }
              frame #1 {
                n73 = Wait (ms)(milliseconds to wait=u32 2000 ("等待时间（毫秒）")) -> ()  [unwired: 1 out]
              }
            }
          }
          frame Error {
          }
        }
        n74 = call "Add State to Queue.vi"("State(s) In Front (\"\")"=w122, "State(s) In (\"\")"=w124) -> ("States Out"=w123:string)  [unwired: 13 in]
      }
      frame "Cal: Calibration failed" {
        n75 = global read "多参数全局变量.vi" "多参数编号"() -> (w141:string)
        n76 = call "Add State to Queue.vi"("State(s) In (\"\")"="init: all\nCal: Over\nidle" ("State(s) In (\"\")")) -> ("States Out"=w144:string)  [unwired: 14 in]
        n77 = Format Into String(format string="编号：%s\n参数：%s\n信息：%s" ("格式字符串"), w141, w138, "校准失败！" ("消息")) -> (resulting string=w140:string)  [unwired: 2 in, 1 out]
        n78 = One Button Dialog(message=w140) -> ()  [unwired: 1 in, 1 out]
        n79 = call "校准日志.vi"("table"="校准记录", "日志信息"=w140) -> ()  [unwired: 9 in, 1 out]
      }
      frame "Cal: Pass" {
        n80 = flat-sequence {
          tunnel: [w164] -> w151
          frame #0 {
            n81 = Wait (ms)(milliseconds to wait=u32 3000 ("等待时间（毫秒）")) -> ()  [unwired: 1 out]
          }
          frame #1 {
            n82 = local read "第一点校准值"() -> (w163:dbl)
            n83 = local read "第一点信号值"() -> (w161:dbl)
            n84 = local read "标液1"() -> (w160:dbl)
            n85 = Format Into String(format string="校准结果：\n校准值=%#.2f，信号值=%#.2f，标准值=%#.2f。" ("提示"), w163, w161, w160) -> (resulting string=w164:string)  [unwired: 2 in, 1 out]
          }
        }
        n86 = call "Add State to Queue.vi"("State(s) In (\"\")"="init: all\nCal: Over\nidle" ("State(s) In (\"\")")) -> ("States Out"=w149:string)  [unwired: 14 in]
        n87 = global read "多参数全局变量.vi" "多参数编号"() -> (w155:string)
        n88 = Format Into String(format string="编号：%s\n参数：%s\n信息：%s" ("格式字符串"), w155, w154, w151) -> (resulting string=w152:string)  [unwired: 2 in, 1 out]
        n89 = One Button Dialog(message=w152) -> ()  [unwired: 1 in, 1 out]
        n90 = call "校准日志.vi"("table"="校准记录", "日志信息"=w152) -> ()  [unwired: 9 in, 1 out]
      }
      frame "Cal: Over" {
        n91 = global read "多参数全局变量.vi" "校准运行状态"() -> (w170:T7)
        n92 = Bundle By Name(cluster=w170, "ORP"=FALSE) -> (w171:T7)
        n93 = global write "多参数全局变量.vi" "校准运行状态"(w171) -> ()
      }
      frame "idle", Default {
        n94 = event shown="[5] \"滤波设定\": 值改变" {
          selector: _ -> [_ _ _ _ _ _ _ _ _]
          dyn-events: _ -> [_ _ _ _ _ _ _ _ _]
          timeout: 10 -> [_ _ _ _ _ _ _ _ _]
          tunnel: [_ _ _ _ w211 w221 _ _ _] -> _
          tunnel: w179 -> [w192 w196 w201 _ w218 w228 w235 _ _]
          tunnel: [w191 w195 w203 w205 w217 w227 w234 w237 w240] -> w178
          tunnel: [w190 w193 w204 w207 w216 w226 w232 w238 w239] -> w177
          tunnel: w176 -> [w190 w193 w204 w207 w216 w226 w232 w238 w239]
          tunnel: w172 -> [_ _ _ _ w210 w220 _ _ _]
          event Timeout {
            n95 = event-data() -> ()  [unwired: 1 in, 3 out]
            n96 = global read "多参数全局变量.vi" "orp通讯状态"() -> (w188:bool)
            n97 = property on="通讯状态" class="Str"("Blinking"=TRUE ("闪烁"), "Text.BG Color"=u32 16711680, "Visible"=w188) -> ()  [unwired: 2 in, 2 out]
            n98 = global read "国弘过程全局变量.vi" "ORP"() -> (w181:T4)
            n99 = Unbundle By Name(w181) -> ("命令滤波设定"=→"滤波设定":u16, "偏移修正值"=→"ORP偏移修正值":sgl, "测量值"=→"当前读取值":sgl, "信号值"=→"当前信号值":sgl, "温度测量值"=→"温度":sgl)  [unwired: 1 out]
            n100 = call "Add State to Queue.vi"("State(s) In (\"\")"=w192) -> ("States Out"=w191:string)  [unwired: 14 in]
            "通讯状态" <- "通讯异常" ("当前串口")
          }
          event "校准模式": Value Change {
            n101 = event-data() -> ()  [unwired: 1 in, 6 out]
            n102 = call "Add State to Queue.vi"("State(s) In (\"\")"=w196, "State(s) At Back (\"\")"="init: all\nidle" ("State(s) In (\"\")")) -> ("States Out"=w195:string)  [unwired: 13 in]
          }
          event "标液1", "ORP偏移修正值": Mouse Down {
            n103 = event-data() -> ("CtlRef"=w200:refnum<vi>)  [unwired: 1 in, 7 out]
            n104 = property class="DigNum (严格)"(reference=w200) -> (reference out=w197:refnum<vi>, "Value"=w198:dbl)  [unwired: 1 in, 1 out]
            n105 = call "数字键盘.vi"("OldNumber"=w198) -> ("NewNumber"=w199:dbl)  [unwired: 1 in]
            n106 = property class="DigNum (严格)"(reference=w197, "Val(Sgnl)"=w199) -> ()  [unwired: 1 in, 2 out]
            n107 = call "Add State to Queue.vi"("State(s) In (\"\")"=w201, "State(s) At Back (\"\")"="idle" ("State(s) In (\"\")")) -> ("States Out"=w203:string)  [unwired: 13 in]
          }
          event "标液1": Value Change {
            n108 = event-data() -> ()  [unwired: 1 in, 6 out]
            n109 = flat-sequence {
              frame #0 {
                n110 = global write "断电保存变量.vi" "orp标液1"("标液1") -> ()
              }
              frame #1 {
                n111 = call "配置文件保存.vi"() -> ()  [unwired: 12 in]
              }
            }
            n112 = call "Add State to Queue.vi"("State(s) In (\"\")"="idle" ("State(s) In (\"\")")) -> ("States Out"=w205:string)  [unwired: 14 in]
          }
          event "ORP偏移修正值": Value Change {
            n113 = event-data() -> ("NewVal"=w212:dbl)  [unwired: 1 in, 5 out]
            n114 = global read "多参数全局变量.vi" "MB session in"() -> (w214:refnum<class "MB_Master.lvclass">)
            n115 = call "000CH_ORP_ORP偏移修正值写入.vi"("数值"=w212, "MB session in"=w214) -> ("error out"=w213:errorcluster)  [unwired: 8 in, 1 out]
            n116 = Enqueue Element At Opposite End(queue=w210, element=T5."ORP" ("元素"), error in (no error)=w213) -> (error out=w211:errorcluster)  [unwired: 1 in, 2 out]
            n117 = call "Add State to Queue.vi"("State(s) In (\"\")"=w218, "State(s) At Back (\"\")"="idle" ("State(s) In (\"\")")) -> ("States Out"=w217:string)  [unwired: 13 in]
          }
          event "滤波设定": Value Change {
            n118 = event-data() -> ("NewVal"=w223:dbl)  [unwired: 1 in, 5 out]
            n119 = global read "多参数全局变量.vi" "MB session in"() -> (w224:refnum<class "MB_Master.lvclass">)
            n120 = call "0027H_ORP_数位滤波设定写入.vi"("数值"=w223, "MB session in"=w224) -> ("error out"=w222:errorcluster)  [unwired: 8 in, 1 out]
            n121 = Enqueue Element At Opposite End(queue=w220, element=T5."ORP" ("元素"), error in (no error)=w222) -> (error out=w221:errorcluster)  [unwired: 1 in, 2 out]
            n122 = call "Add State to Queue.vi"("State(s) In (\"\")"=w228, "State(s) At Back (\"\")"="idle" ("State(s) In (\"\")")) -> ("States Out"=w227:string)  [unwired: 13 in]
          }
          event "校准启动": Value Change {
            n123 = event-data() -> ()  [unwired: 1 in, 6 out]
            n124 = global read "多参数全局变量.vi" "校准运行状态"() -> (w230:T7)
            n125 = call "Add State to Queue.vi"("State(s) In (\"\")"=w235, "State(s) At Back (\"\")"="init: all\nCal: Place standard solution\n Cal: Calibration process\nidle" ("State(s) In (\"\")")) -> ("States Out"=w234:string)  [unwired: 13 in]
            n126 = Bundle By Name(cluster=w230, "ORP"=TRUE) -> (w231:T7)
            n127 = global write "多参数全局变量.vi" "校准运行状态"(w231) -> ()
          }
          event "校准停止": Value Change {
            n128 = event-data() -> ()  [unwired: 1 in, 6 out]
            n129 = call "Add State to Queue.vi"("State(s) In (\"\")"="init: all\nCal: Over\nidle" ("State(s) In (\"\")")) -> ("States Out"=w237:string)  [unwired: 14 in]
          }
          event "刷新按钮": Value Change {
            n130 = event-data() -> ()  [unwired: 1 in, 6 out]
            n131 = Two Button Dialog(message="请再次确实是否恢复出厂设置！" ("消息")) -> (T button?=w243:bool)  [unwired: 2 in]
            n132 = case shown="真" w243 {
              frame False {
              }
              frame True {
                w244 = u16 33 items=["Factory Reset"=33] ("数值")
                n133 = global read "多参数全局变量.vi" "MB session in"() -> (w245:refnum<class "MB_Master.lvclass">)
                n134 = call "0026H_ORP_命令寄存器写入.vi"("数值"=w244, "MB session in"=w245) -> ()  [unwired: 8 in, 2 out]
              }
            }
            n135 = call "Add State to Queue.vi"("State(s) In (\"\")"="init: all\nidle" ("State(s) In (\"\")")) -> ("States Out"=w240:string)  [unwired: 14 in]
          }
        }
      }
    }
  }
  n136 = while {
    stop <- FALSE stop-if-true
    n137 = global read "多参数全局变量.vi" "权限"() -> (w249:enum16{"一级权限", "二级权限", "三级权限"})
    n138 = Wait (ms)(milliseconds to wait=u32 1000 ("等待时间（毫秒）")) -> ()  [unwired: 1 out]
    n139 = Not Equal?(x=w249, y=enum16{"一级权限", "二级权限", "三级权限"}."一级权限") -> (x != y?=w246:bool)
    n140 = property on="滤波设定" class="DigNum (严格)"("Visible"=w246) -> ()  [unwired: 2 in, 2 out]
    n141 = property on="ORP偏移修正值" class="DigNum (严格)"("Visible"=w246) -> ()  [unwired: 2 in, 2 out]
  }
